vi "Clear Range.vi"(8 "error in (no error)":errorcluster, 9 "end position (end of line)":cluster{"row":i8, "column":i8}={"row"=-1, "column"=-1}, 10 "start position":cluster{"row":i8, "column":i8}, 11 "LCD in":refnum<class "Character LCD.lvclass">) -> (0 "error out":errorcluster, 3 "LCD out":refnum<class "Character LCD.lvclass">)   [LabVIEW 2017, in "HD44780 Host.lvlib"]
doc: "Clears a continuous area on the display of LCD devices.\n\nORIGINAL CODE: \nBy: National Instruments\n NI LabVIEW RIO Evaluation Kit\n Code example \"5- Startup Application\"\n www.ni.com/embeddedsystems\n\nUPDATED CODE: Adds NI SystemLink and NI AWS LabVIEW Tookit functionality for demonstration. \nBy: James Tillett\n Endeavor Engineering Inc.\n www.endeavoreng.com"
uses:
  HD44780 Host.lvlib
  Internal/LCD Class/Character LCD.lvclass
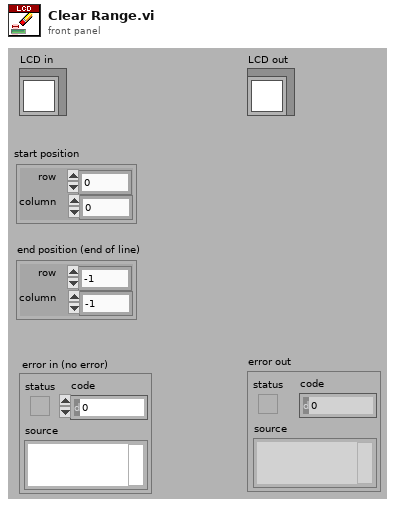
[diagram p1: front panel]
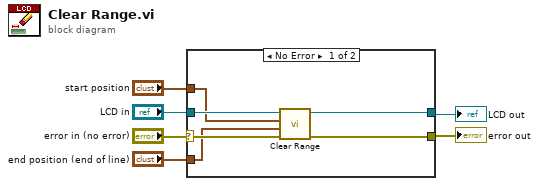
[diagram p0: block diagram]
diagram:
  n1 = case shown="No Error" "error in (no error)" {
    selector: "error in (no error)" -> [w9 w14]
    tunnel: [w10 w14] -> w5
    tunnel: "LCD in" -> [w12 w13]
    tunnel: [w11 w13] -> w3
    tunnel: "end position (end of line)" -> [w8 _]
    tunnel: "start position" -> [w7 _]
    frame No Error {
      n2 = call-dynamic "Clear Range.vi"("error in (no error)"=w9, "end position (end of line)"=w8, "start position"=w7, "Character LCD in"=w12) -> ("error out"=w10:errorcluster, "Character LCD out"=w11:refnum<class "Character LCD.lvclass">)  [unwired: 6 in]
    }
    frame Error {
    }
  }
  "error out" <- w5
  "LCD out" <- w3
